vi "Multi-Table Insert.vi"(5 "Columns of insert for  Table 1":string, 6 "Table 2 column 2":string, 7 "Table 1 data":string, 8 "error in":errorcluster, 9 "Table 1 path":string, 10 "Table 2 path":string, 11 "LV-Data.PGSQL":refnum<class "LV-Data.PGSQL.lvclass">) -> (0 "error out":errorcluster, 3 "LV-Data.PGSQL out":refnum<class "LV-Data.PGSQL.lvclass">)   [LabVIEW 2016, in "LV-Data.PGSQL.lvclass"]
uses:
  LV-Data.PGSQL.lvclass
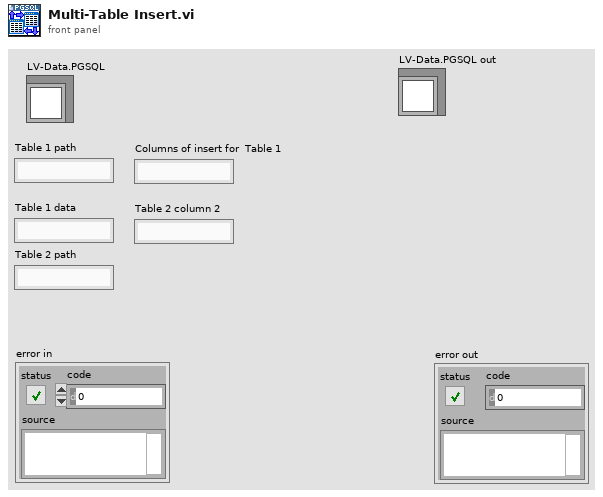
[diagram p1: front panel]
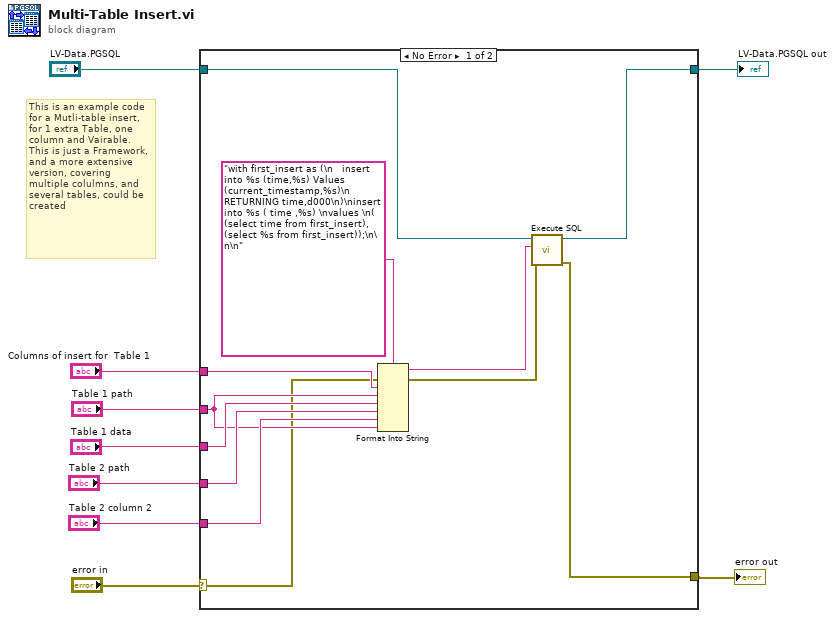
[diagram p0: block diagram]
diagram:
  # "This is an example code for a Mutli-table insert, for 1 extra Table, one column and Vairable. \nThis is just a Framework, and a more extensive version, covering multiple colulmns, and several tables, could be created"
  n1 = case shown="No Error" "error in" {
    selector: "error in" -> [w14 w22]
    tunnel: "Columns of insert for  Table 1" -> [w20 _]
    tunnel: "Table 1 path" -> [w16 _]
    tunnel: "Table 1 data" -> [w19 _]
    tunnel: "Table 2 path" -> [w18 _]
    tunnel: "Table 2 column 2" -> [w17 _]
    tunnel: [w12 w22] -> w3
    tunnel: "LV-Data.PGSQL" -> [w11 w23]
    tunnel: [w10 w23] -> w1
    frame No Error {
      n2 = Format Into String(format string="with first_insert as (\n   insert into %s (time,%s) Values (current_timestamp,%s)\n   RETURNING time,d000\n)\ninsert into %s ( time ,%s) \nvalues \n( (select time from first_insert), (select %s from first_insert));\n\n\n", error in=w14, w20, w16, w19, w18, w17, w16) -> (resulting string=w15:string, error out=w13:errorcluster)  [unwired: 1 in]
      n3 = call "Execute SQL.vi"("error in"=w13, "SQL"=w15, "LV-Data.PGSQL"=w11) -> ("error out"=w12:errorcluster, "LV-Data.PGSQL out"=w10:refnum<class "LV-Data.PGSQL.lvclass">)  [unwired: 6 in, 1 out]
    }
    frame Error {
    }
  }
  "error out" <- w3
  "LV-Data.PGSQL out" <- w1
